vi "向量求解.vi"() -> ()   [LabVIEW 2018]
uses:
  <vilib>/Analysis/Matrix/Datatypes/RealMatrix.ctl
  <vilib>/Analysis/7linalg.llb/Solve Linear Equations (single right hand).vi
  <vilib>/Analysis/baseanly.llb/Solve Linear Equations By Cholesky.vi
  <vilib>/Analysis/baseanly.llb/Real Matrix to Compact Array.vi
  <vilib>/Analysis/baseanly.llb/Real Compact Tri-Matrix Linear Eqs.vi
  <vilib>/Analysis/7linalg.llb/Solve Linear Eqs (General).vi
  <vilib>/Analysis/7linalg.llb/Solve Linear Eqs (Gen, single right hand).vi
  <vilib>/Analysis/NI_AALPro.lvlib
  <vilib>/Analysis/Matrix/NI_Matrix.lvlib
panel:
  in  "停止":bool
  out "Solution Vector":dbl[](array[numeric]) caption="向量解" format="%.2f"
  in  "B":dbl[](array[numeric]) caption="右端项" format="%.2f"
  in  "A":T1 caption="输入矩阵"
  # "X"
  # "="
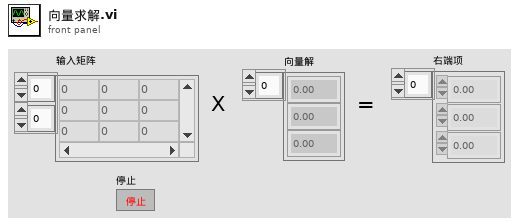
[diagram p1: front panel]
types:
  T1 = typedef "NI_Matrix.lvlib/RealMatrix.ctl" = dbl[][]
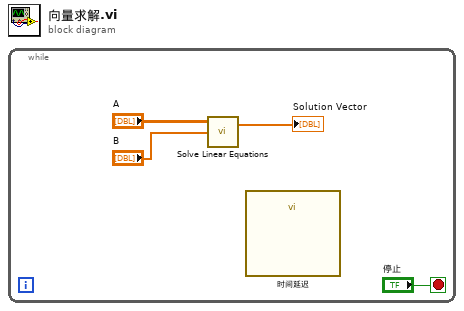
[diagram p0: block diagram]
diagram:
  n1 = while {
    stop <- "停止" stop-if-true
    n2 = call-poly <vilib>:"Solve Linear Equations.vi"("Known Vector"="B", "Input Matrix"="A") -> ("Solution Vector"=→"Solution Vector":dbl[])  [unwired: 1 in, 1 out]
    n3 = call "时间延迟"() -> ()  [unwired: 11 in, 1 out]
  }
